vi "TestExec.Split ScriptCmd Name to Module and Funct.vi"(10 "Cmd":string, 11 "Modules":string[](array[string])) -> (1 "Found":bool, 2 "Cmd":string, 3 "Module":string)   [LabVIEW 2019]
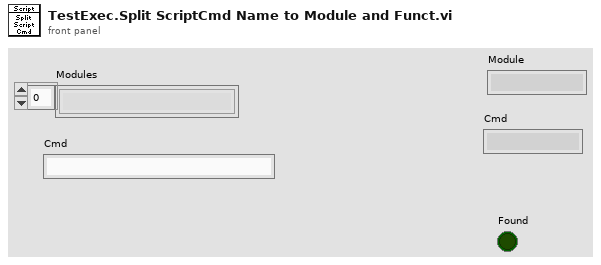
[diagram p1: front panel]
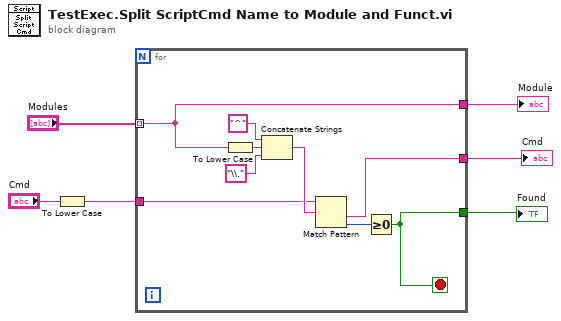
[diagram p0: block diagram]
diagram:
  n1 = To Lower Case(string="Cmd") -> (all lower case string=w6:string)
  n2 = for {
    tunnel: w6 -> [w10]
    tunnel: [w9] -> w4
    tunnel: "Modules" -> [w8] mode=indexing
    tunnel: [w8] -> w2
    tunnel: [w7] -> w1
    stop <- w9 stop-if-true
    n3 = To Lower Case(string=w8) -> (all lower case string=w14:string)
    n4 = Concatenate Strings("^", w14, "\\.") -> (w12:string)
    n5 = Match Pattern(string=w10, regular expression=w12) -> (after substring=w7:string, offset past match=w11:i32)  [unwired: 1 in, 2 out]
    n6 = Greater Or Equal To 0?(x=w11) -> (x >= 0?=w9:bool)
  }
  "Found" <- w4
  "Module" <- w2
  "Cmd" <- w1
